vi "generate structural test.vi"(8 "error in (no error)":errorcluster, 11 "Tdms File":refnum<k34>) -> (0 "error out":errorcluster, 3 "Tdms File Out":refnum<k34>)   [LabVIEW 2020]
doc: "Writes alternating segments of 2 sets of channels in the same group. ch1-3 at 1000 per write and 4-6 at 500 per write.\n\nEach pair of writes is alternated between interleaved and decimated data."
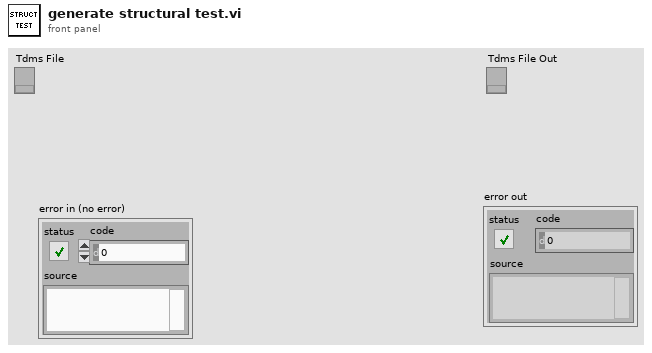
[diagram p1: front panel]
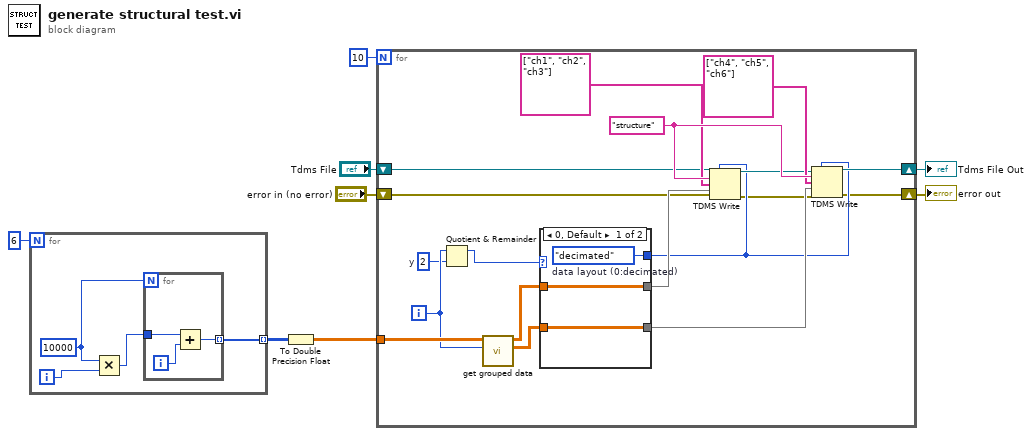
[diagram p0: block diagram]
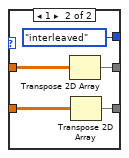
[diagram p2: hidden frame]
diagram:
  n1 = for {
    N: 6 -> [_]
    tunnel: [w10] -> w7 mode=indexing
    i -> [w12]
    w9 = 10000 ("x")
    n2 = Multiply(x=w9, y=w12) -> (x*y=w11:i32)
    n3 = for {
      N: w9 -> [_]
      tunnel: w11 -> [w14]
      tunnel: [w13] -> w10 mode=indexing
      i -> [w15]
      n4 = Add(x=w14, y=w15) -> (x+y=w13:i32)
    }
  }
  n5 = To Double Precision Float(number=w7) -> (double precision float=w5:dbl[][])
  n6 = for {
    N: 10 -> [_]
    tunnel: w5 -> [w33]
    shift-right: [w27] -> w3
    shift-left: "Tdms File" -> [w26]
    shift-right: [w17] -> w1
    shift-left: "error in (no error)" -> [w16]
    i -> [w24]
    w23 = 2  # y
    w32 = "structure" ("group name in (Untitled)")
    n7 = Quotient & Remainder(x=w24, y=w23) -> (x-y*floor(x/y)=w19:i32)  [unwired: 1 out]
    n8 = call "get grouped data.vi"("Index"=w24, "Full Data Set"=w33) -> ("Small Group"=w28:dbl[][], "Large Group"=w29:dbl[][])  [unwired: 8 in]
    n9 = case shown="0, Default" w19 {
      tunnel: w29 -> [w35 w41]
      tunnel: w28 -> [w34 w40]
      tunnel: [w35 w39] -> w22
      tunnel: [w34 w38] -> w21
      tunnel: [w36 enum16{"decimated", "interleaved"}."interleaved" ("data layout (0:decimated)")] -> w20
      frame 0, Default {
        w36 = enum16{"decimated", "interleaved"}."decimated"  # data layout (0:decimated)
      }
      frame 1 {
        n10 = Transpose 2D Array(2D array=w41) -> (transposed array=w39:dbl[][])
        n11 = Transpose 2D Array(2D array=w40) -> (transposed array=w38:dbl[][])
      }
    }
    n12 = TDMS Write(0:w26, 1:w20, 5:w32, 7:string[] ["ch1", "ch2", "ch3"] ("channel name(s) in (Untitled)"), 9:w22, 11:w16) -> (4:w25:refnum<k34>, 15:w18:errorcluster)  [unwired: 2 out]
    n13 = TDMS Write(0:w25, 1:w20, 5:w32, 7:string[] ["ch4", "ch5", "ch6"] ("channel name(s) in (Untitled)"), 9:w21, 11:w18) -> (4:w27:refnum<k34>, 15:w17:errorcluster)  [unwired: 2 out]
  }
  "Tdms File Out" <- w3
  "error out" <- w1
